vi "test Set Routing Channel State Configurations Updates State Value Table.vi"(8 "error in (no error)":errorcluster, 11 "TestCase in":refnum<class "Routing and Faulting Scripting Unit Tests.lvclass">) -> (0 "error out":errorcluster, 3 "TestCase out":refnum<class "Routing and Faulting Scripting Unit Tests.lvclass">)   [LabVIEW 2017, in "Routing and Faulting Scripting Unit Tests.lvclass"]
uses:
  Routing and Faulting Scripting Unit Tests.lvclass
  Shared/Channel States.ctl
  Shared/Routing State.ctl
  Shared/Connection.ctl
  Routing and Faulting Scripting Unit Tests.lvclass/Routing and Faulting Scripting Unit Tests.ctl
  <vilib>/addons/_JKI Toolkits/VI Tester/TestCase.llb/TestCase.lvclass
  Routing and Faulting Scripting.lvlib
  Shared/Routing and Faulting Shared.lvlib
  C:/Program Files (x86)/National Instruments/LabVIEW 2017/vi.lib/addons/_JKI Toolkits/VI Tester/TestCase.llb/TestCase.lvclass
panel:
  in  "Save?":bool
  out "Output Filename":string
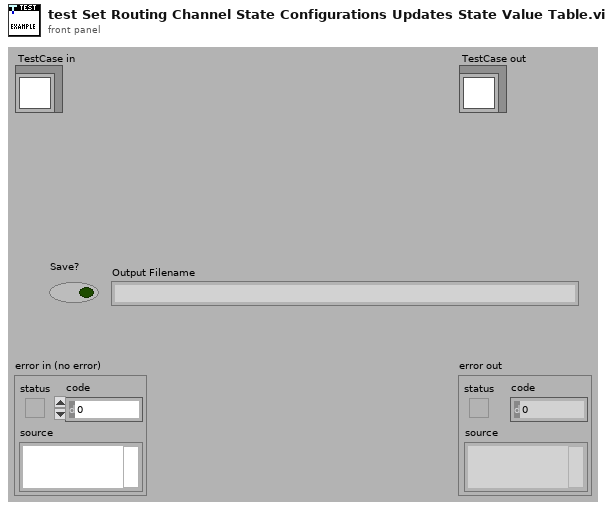
[diagram p1: front panel]
types:
  T1 = typedef "Routing and Faulting Shared.lvlib/Channel States.ctl" = T2[]
  T2 = typedef "Routing and Faulting Shared.lvlib/Routing State.ctl" = cluster{"Name":string, "Description":string, "Value":i32, "Connection List":T3[]}
  T3 = typedef "Routing and Faulting Shared.lvlib/Connection.ctl" = cluster{"Module":string, "Source":string, "Destination":string}
  T4 = typedef "Custom Device API.lvlib/Custom Device Item Ref.ctl" = u64
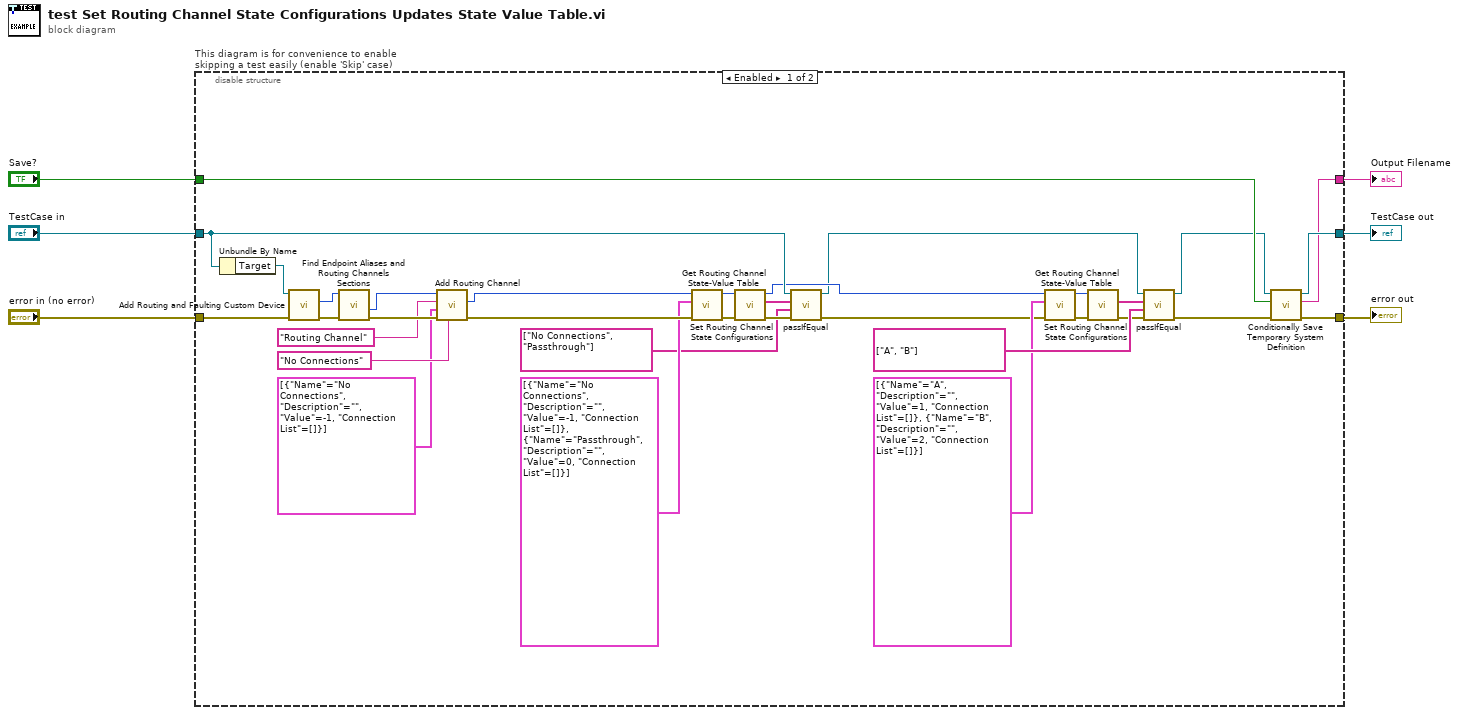
[diagram p0: block diagram]
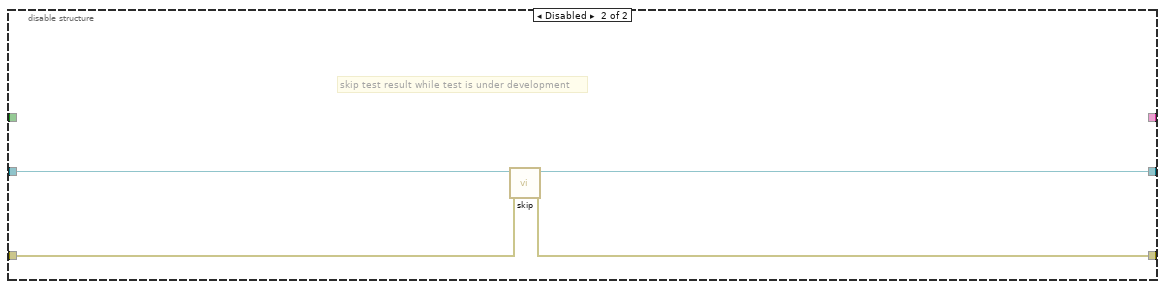
[diagram p2: hidden frame]
diagram:
  n1 = disable-structure "This diagram is for convenience to enable skipping a test easily (enable 'Skip' case)" shown="Enabled" {
    disable-tunnel: "TestCase in" -> [w20 w43]
    disable-tunnel: [w28 w41] -> w3
    disable-tunnel: [w29 w42] -> w5
    disable-tunnel: "error in (no error)" -> [w34 w40]
    disable-tunnel: "Save?" -> [w27 _]
    disable-tunnel: [w26 _] -> w1
    frame Enabled {
      n2 = Unbundle By Name(w20) -> ("Target"=w39:refnum<k24>)
      n3 = call "Add Routing and Faulting Custom Device.vi"("error in"=w34, "target in"=w39) -> ("error out"=w38:errorcluster, "routing and faulting custom device"=w37:T4)  [unwired: 7 in, 1 out]
      n4 = call "Find Endpoint Aliases and Routing Channels Sections.vi"("error in"=w38, "routing and faulting custom device in"=w37) -> ("error out"=w36:errorcluster, "routing channels"=w35:T4)  [unwired: 6 in, 2 out]
      n5 = call "Add Routing Channel.vi"("initial state"="No Connections", "error in"=w36, "state configurations"=T1 [{"Name"="No Connections", "Description"="", "Value"=-1, "Connection List"=[]}], "channel name"="Routing Channel", "routing channels in"=w35) -> ("error out"=w30:errorcluster, "routing channel"=w24:T4)  [unwired: 4 in, 1 out]
      n6 = call "Set Routing Channel State Configurations.vi"("error in"=w30, "state configurations"=T1 [{"Name"="No Connections", "Description"="", "Value"=-1, "Connection List"=[]}, {"Name"="Passthrough", "Description"="", "Value"=0, "Connection List"=[]}], "routing channel in"=w24) -> ("error out"=w25:errorcluster, "routing channel out"=w22:T4)  [unwired: 7 in]
      n7 = call "Get Routing Channel State-Value Table.vi"("error in"=w25, "routing channel in"=w22) -> ("error out"=w21:errorcluster, "state names"=w19:string[], "routing channel out"=w9:T4)  [unwired: 6 in, 1 out]
      n8 = call-dynamic "passIfEqual.vi"("error in (no error)"=w21, "y"=string[] ["No Connections", "Passthrough"] ("state names"), "x"=w19, "TestCase in"=w20) -> ("error out"=w10:errorcluster, "TestCase out"=w8:refnum<class "Routing and Faulting Scripting Unit Tests.lvclass">)  [unwired: 6 in]
      n9 = call "Set Routing Channel State Configurations.vi"("error in"=w10, "state configurations"=T1 [{"Name"="A", "Description"="", "Value"=1, "Connection List"=[]}, {"Name"="B", "Description"="", "Value"=2, "Connection List"=[]}], "routing channel in"=w9) -> ("error out"=w12:errorcluster, "routing channel out"=w14:T4)  [unwired: 7 in]
      n10 = call "Get Routing Channel State-Value Table.vi"("error in"=w12, "routing channel in"=w14) -> ("error out"=w15:errorcluster, "state names"=w16:string[])  [unwired: 6 in, 2 out]
      n11 = call-dynamic "passIfEqual.vi"("error in (no error)"=w15, "y"=string[] ["A", "B"] ("state names"), "x"=w16, "TestCase in"=w8) -> ("error out"=w11:errorcluster, "TestCase out"=w7:refnum<class "Routing and Faulting Scripting Unit Tests.lvclass">)  [unwired: 6 in]
      n12 = call "Conditionally Save Temporary System Definition.vi"("error in (no error)"=w11, "Save?"=w27, "Test Case"=w7) -> ("error out"=w29:errorcluster, "filename"=w26:string, "Test Case"=w28:refnum<class "Routing and Faulting Scripting Unit Tests.lvclass">)  [unwired: 6 in]
    }
    frame Disabled {
      # "skip test result while test is under development"
      n13 = call <vilib>:"skip.vi"("error in (no error)"=w40, "TestCase in"=w43) -> ("error out"=w42:errorcluster, "TestCase out"=w41:refnum<class "Routing and Faulting Scripting Unit Tests.lvclass">)  [unwired: 8 in]
    }
  }
  "error out" <- w5
  "TestCase out" <- w3
  "Output Filename" <- w1
